vi "Log Data to File.vi"(8 "error in (no error)":errorcluster, 10 "Data to log":waveform(dbl)[](array[waveform]), 11 "TDMS File Reference":refnum<k34>) -> (0 "error out":errorcluster)   [LabVIEW 2019, in "Logger.lvlib"]
doc: "This VI uses the TDMS Write function to write data to a TDMS file.\n_____\nBased on Delacor QMH Project Template 5.0.0.82."
uses:
  Logger.lvlib
  <vilib>/Utility/file.llb/Write Delimited Spreadsheet (DBL).vi
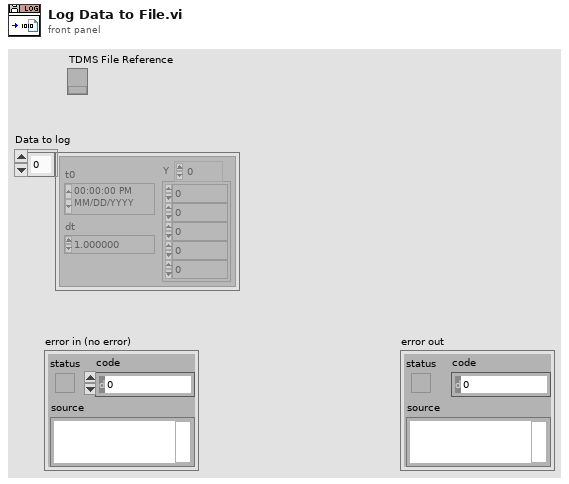
[diagram p1: front panel]
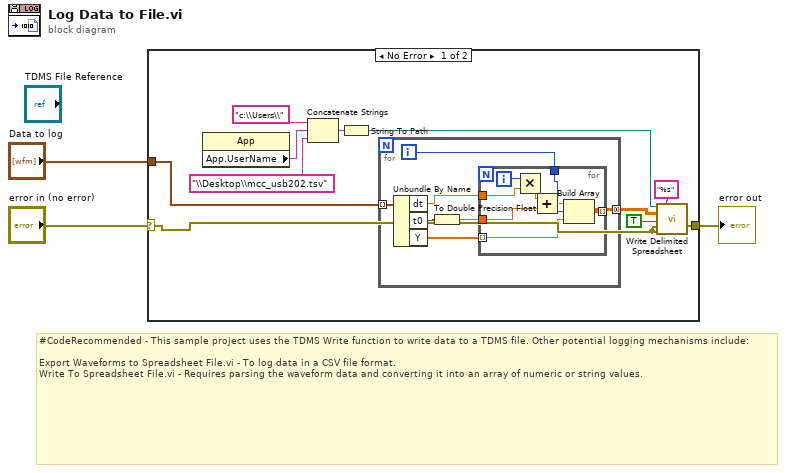
[diagram p0: block diagram]
diagram:
  # "#CodeRecommended - This sample project uses the TDMS Write function to write data to a TDMS file. Other potential logging mechanisms include:\n\nExport Waveforms to Spreadsheet File.vi - To log data in a CSV file format.\nWrite To Spreadsheet File.vi - Requires parsing the waveform data and converting it into an array of numeric or string values."
  n1 = case shown="No Error" "error in (no error)" {
    selector: "error in (no error)" -> [w6 w29]
    tunnel: "Data to log" -> [w5 _]
    tunnel: [w6 w29] -> w2
    frame No Error {
      n2 = property class="App"() -> ("App.UserName"=w12:string)  [unwired: 2 in, 2 out]
      n3 = Concatenate Strings("c:\\Users\\", w12, "\\Desktop\\mcc_usb202.tsv") -> (w10:string)
      n4 = String To Path(string=w10) -> (path=w8:path)
      n5 = for {
        tunnel: w5 -> [w20] mode=indexing
        tunnel: [w19] -> w7 mode=concatenating
        i -> [w17]
        n6 = Unbundle By Name(w20) -> ("dt"=w14:dbl, "t0"=w15:timestamp, "Y"=w16:dbl[])
        n7 = To Double Precision Float(number=w15) -> (double precision float=w18:dbl)
        n8 = for {
          tunnel: [w28] -> w19 mode=indexing
          tunnel: w18 -> [w24]
          tunnel: w17 -> [w27]
          tunnel: w16 -> [w26] mode=indexing
          tunnel: w14 -> [w21]
          i -> [w23]
          n9 = Multiply(x=w23, y=w21) -> (x*y=w22:dbl)
          n10 = Add(x=w22, y=w24) -> (x+y=w25:dbl)
          n11 = Build Array(w25, w27, w26) -> (w28:dbl[])
        }
      }
      n12 = call-poly <vilib>:"Write Delimited Spreadsheet.vi"("file path (dialog if empty)"=w8, "format (%.3f)"="%s", "2D data"=w7, "append to file? (new file:F)"=TRUE, "error in (no error)"=w6) -> ()  [unwired: 9 in, 2 out]
    }
    frame Error {
    }
  }
  "error out" <- w2
